vi "Get SLSC Switch Resource.vi"(8 "error in (no error)":errorcluster, 11 "SLSC Switch Custom Device Ref in":T1 format="%.0x") -> (0 "error out":errorcluster, 2 "Resource":string, 3 "SLSC Switch Custom Device Ref out":T1 format="%.0x")   [LabVIEW 2017, in "SLSC Switch Scripting.lvlib"]
uses:
  SLSC Switch Scripting.lvlib
  <vilib>/NI Veristand/Custom Device API/Custom Device Item Ref.ctl
  Shared/Routing and Faulting Consumer System Definition API/Routing and Faulting Hardware API.lvlib
  <vilib>/NI Veristand/Custom Device API/Custom Device API.lvlib
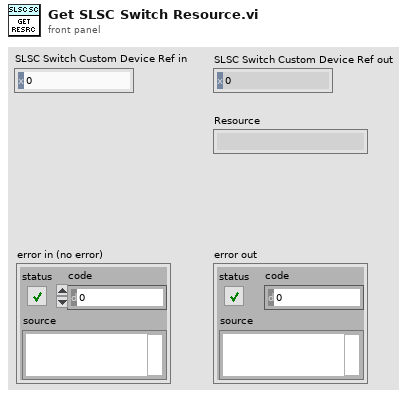
[diagram p1: front panel]
types:
  T1 = typedef "Custom Device API.lvlib/Custom Device Item Ref.ctl" = u64
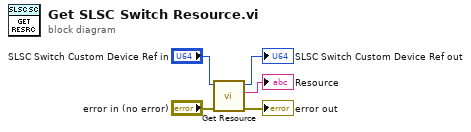
[diagram p0: block diagram]
diagram:
  n1 = call "Get Resource.vi"("error in (no error)"="error in (no error)", "Hardware Ref in"="SLSC Switch Custom Device Ref in") -> ("error out"=→"error out":errorcluster, "Resource"=→"Resource":string, "Hardware Ref out"=→"SLSC Switch Custom Device Ref out":T1)  [unwired: 7 in]
